vi "Create Return FIFO.vi"(8 "error in (no error)":errorcluster, 11 "Transfer Group in":refnum<class "Transfer Group.lvclass">) -> (0 "error out":errorcluster, 3 "Transfer Group out":refnum<class "Transfer Group.lvclass">)   [LabVIEW 2017, in "DSF Core.lvlib" / "Transfer Group.lvclass"]
uses:
  Transfer Group.lvclass
  Transfer Group.lvclass/Transfer Group.ctl
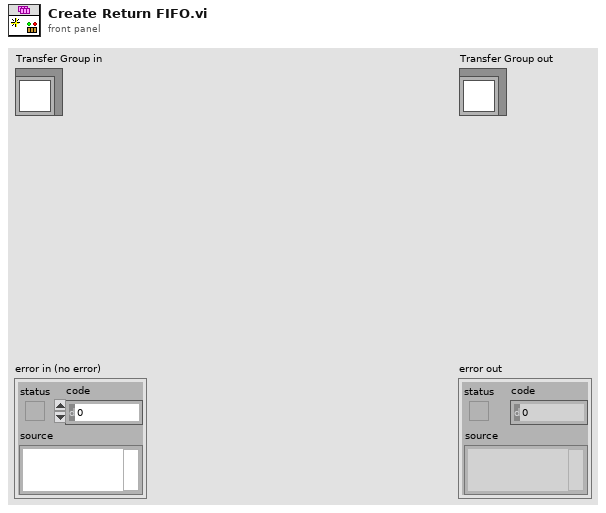
[diagram p1: front panel]
types:
  T1 = cluster{"read mode":enum16{"polling", "blocking"}, "write mode":enum16{"polling", "blocking"}}
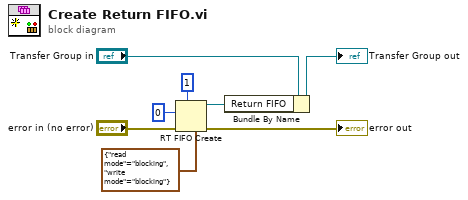
[diagram p0: block diagram]
diagram:
  n1 = RT FIFO Create(1:u64 0, 3:"error in (no error)", 4:u32 1 ("size (10)"), 7:T1 {"read mode"=enum."blocking", "write mode"=enum."blocking"} ("r/w modes (polling,polling)")) -> (8:w3:refnum<k33>, 11:→"error out":errorcluster)  [unwired: 4 in, 1 out]
  n2 = Bundle By Name(cluster="Transfer Group in", "Return FIFO"=w3) -> (→"Transfer Group out":refnum<class "Transfer Group.lvclass">)
